vi "Calibration.vi"(8 "error in (no error)":errorcluster, 11 "Connection Data In":T1) -> (0 "error out":errorcluster={"status"=TRUE, "code"=1172, "source"="Constructor Node Error creating instance of Uri in assembly System.Uri, System, Version=4.0.0.0, Culture=neutral, PublicKeyToken=b77a5c561934e089, (System.UriFormatException: Invalid URI: The hostname could not be parsed.) <append><b>System.UriFormatException</b> in MSX-E3701_dll.lvlib:Connection Open.vi->MSX-E3701_dll.lvlib:Calibration.vi"}, 3 "Connection Data Out":T1)   [LabVIEW 2014, in "MSX-E3711_dll.lvlib"]
doc: "Paanel Frontal que permite la calibracion de transductores."
uses:
  MSX-E3711_dll.lvlib
  Typedef/Calibration Data.ctl
  Typedef/Connection Data.ctl
  E:/Repositorio Magnis/INF002/v0/Modules/HAL/Drivers/Sync/ADDI-DATA MSX-E3711/API/MSXE371x.dll
  MSXE371x.dll
  E:/Repositorio Magnis/INF002/v0/Modules/HAL/Drivers/Sync/ADDI-DATA MSX-E3711/API/MXCommon.dll
  MXCommon.dll
  Typedef/Calibration Enum.ctl
panel:
  out "ulChannel":u64
  in  "Transducer Selection":u64
  in  "Desired Position":dbl format="%#_g[mm]"
  in  "Stop":bool
  out "Progress Bar":u64(slide) scale=0.0..5.0
  out "Measured value":dbl format="%#_g[mm]"
  out "Indicator":string="Leyendo los transductores de la base de datos."
  in  "Next":bool
  in  "Start":bool
  out "Cluster Calibration":T2
  # "TRANSDUCER CALIBRATION"
  # "Progress Bar"
  # "Information"
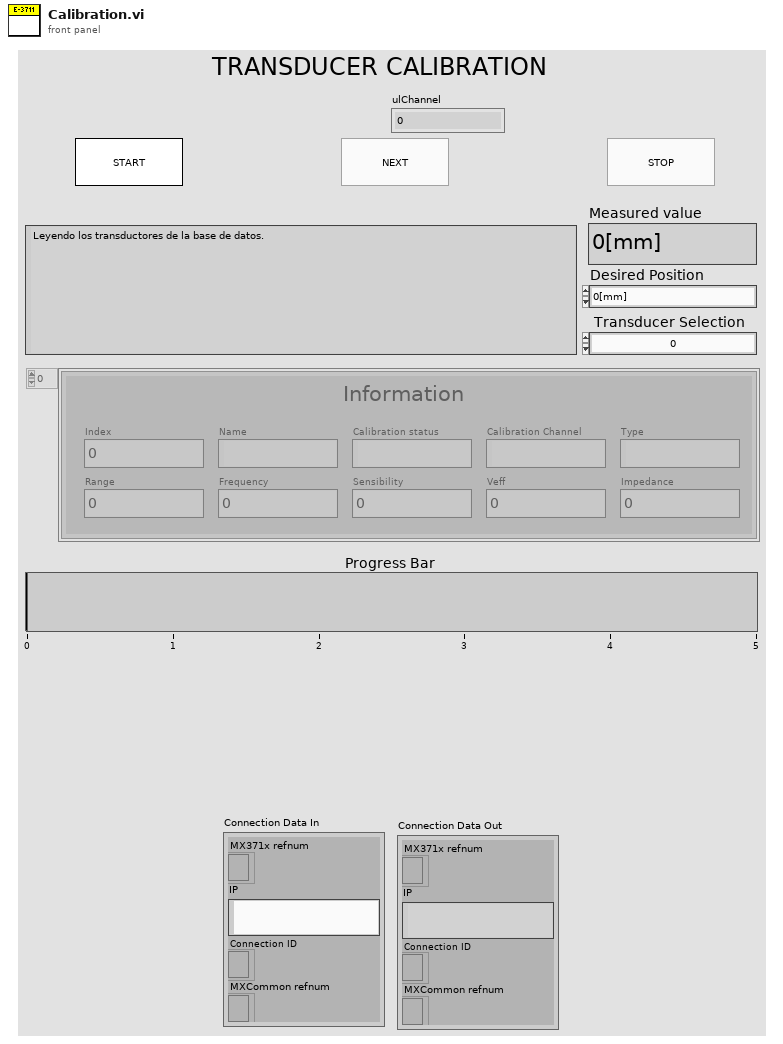
[diagram p1: front panel]
types:
  T1 = typedef "MSX-E3711_dll.lvlib/Connection Data.ctl" = cluster{"MX371x refnum":refnum<k24>, "IP":string, "Connection ID ":refnum<k5>, "MXCommon refnum":refnum<k24>}
  T2 = typedef "MSX-E3711_dll.lvlib/Calibration Data.ctl" = cluster{"Calibration status":string, "Name":string, "Index":u64, "Range":dbl, "Sensibility":dbl, "Veff":dbl, "Frequency":u64, "Impedance":u64, "Type":string, "Calibration Channel":string}[]
  T3 = typedef "MSX-E3711_dll.lvlib/Calibration Enum.ctl" = enum16{"Init", "Idle Start", "Idle Next", "Open Web Service", "Read Transducers", "StartCalibration", "CalibrationGetCurrentStatus", "Save or Omit", "Close Web Service", "Idle Final"}
  T4 = enum8{"Enabled", "Disabled", "Disabled and Grayed Out"}
  T5 = cluster{"Calibration status":string, "Name":string, "Index":u64, "Range":dbl, "Sensibility":dbl, "Veff":dbl, "Frequency":u64, "Impedance":u64, "Type":string, "Calibration Channel":string}
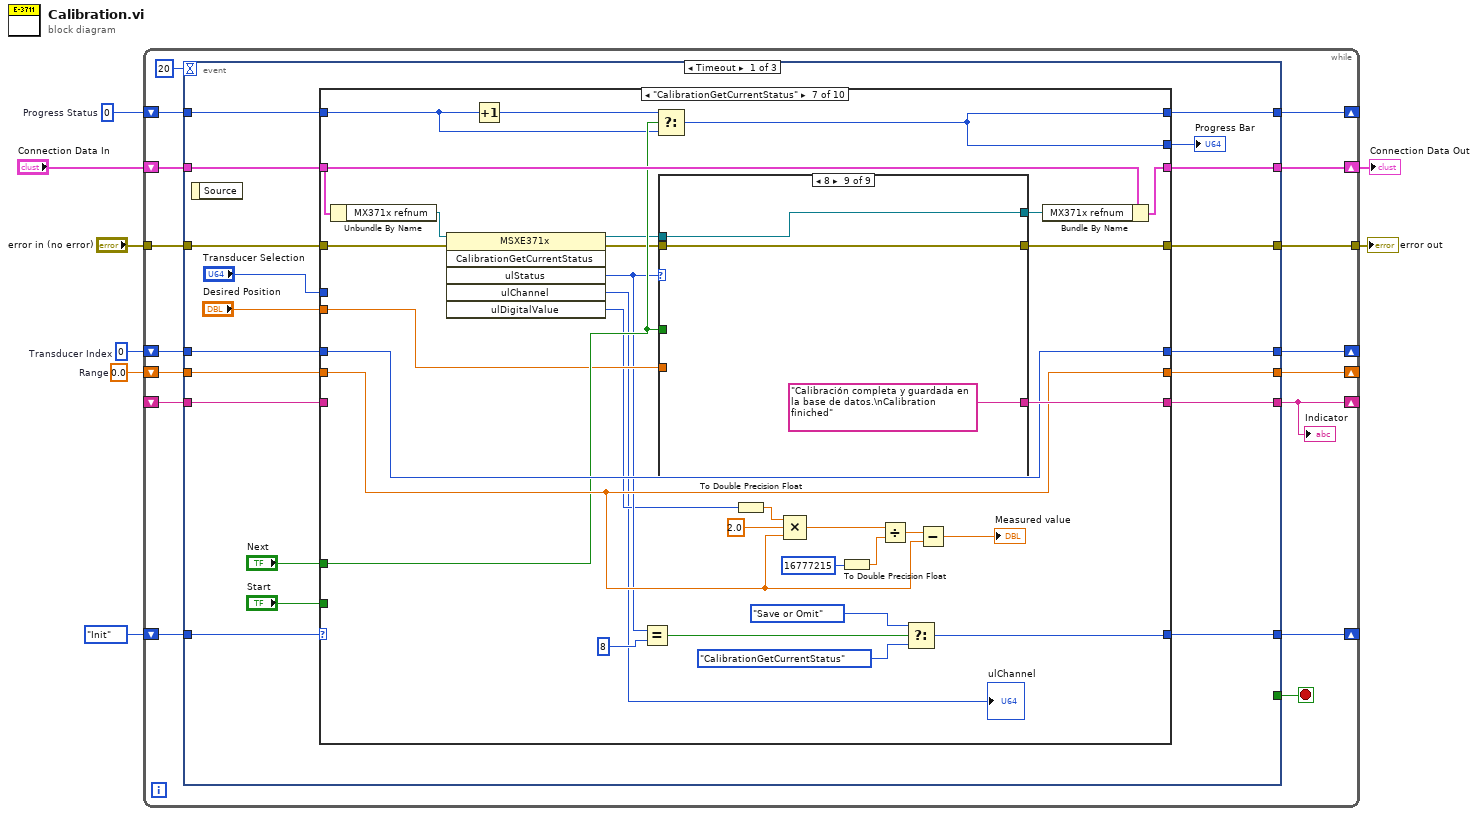
[diagram p0: block diagram]
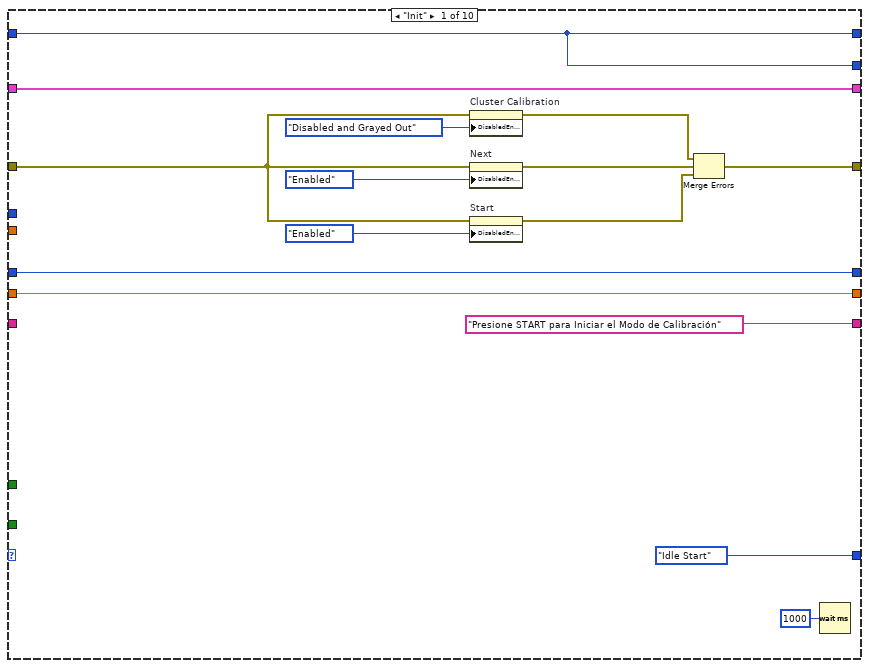
[diagram p2: hidden frame]
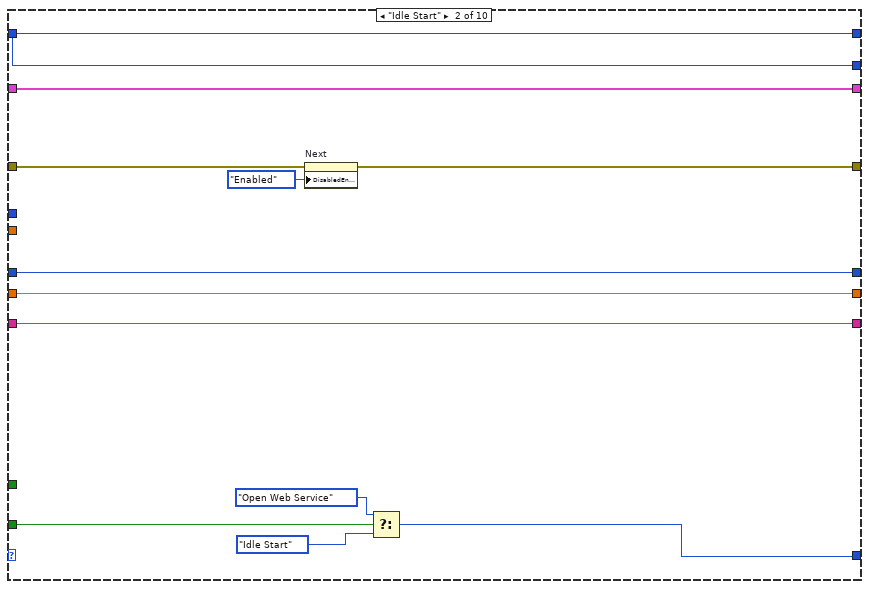
[diagram p3: hidden frame]
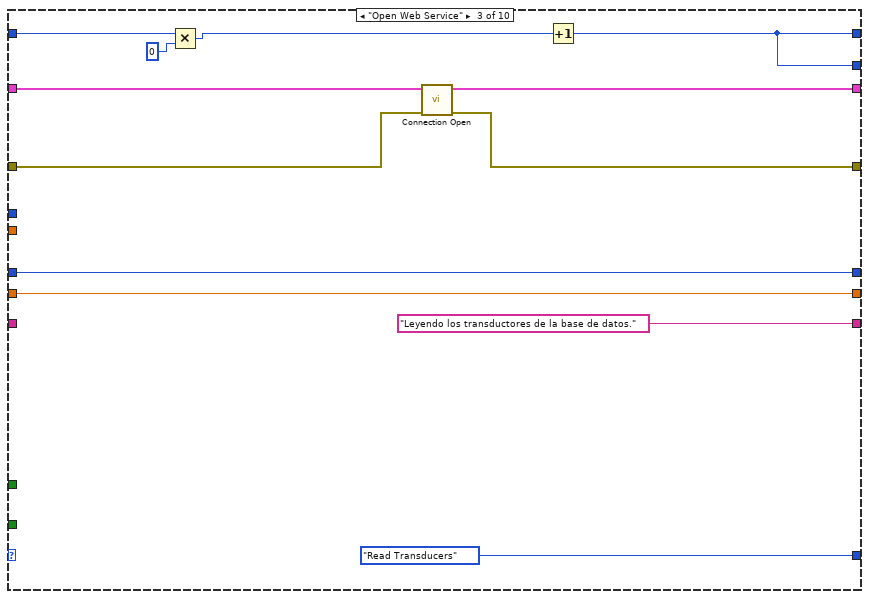
[diagram p4: hidden frame]
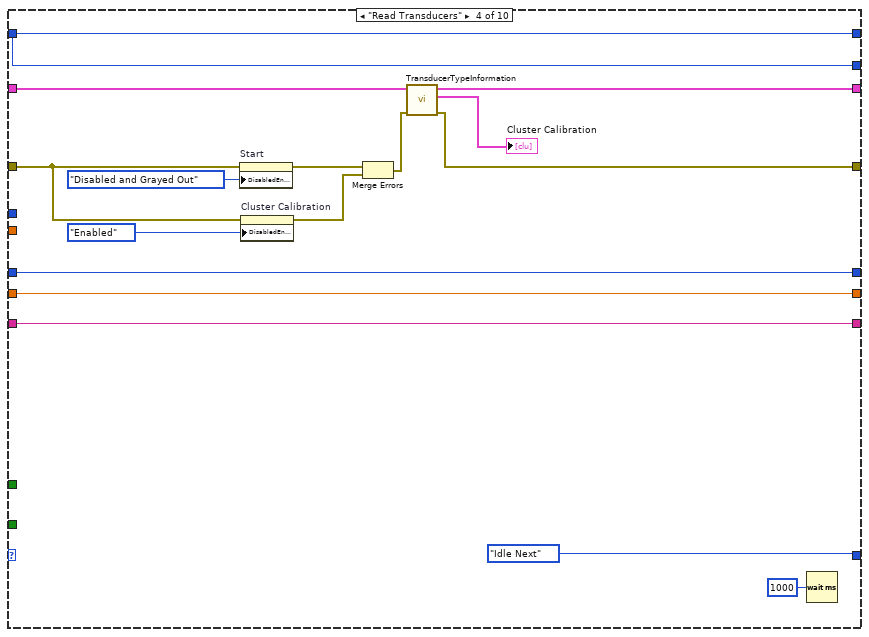
[diagram p5: hidden frame]
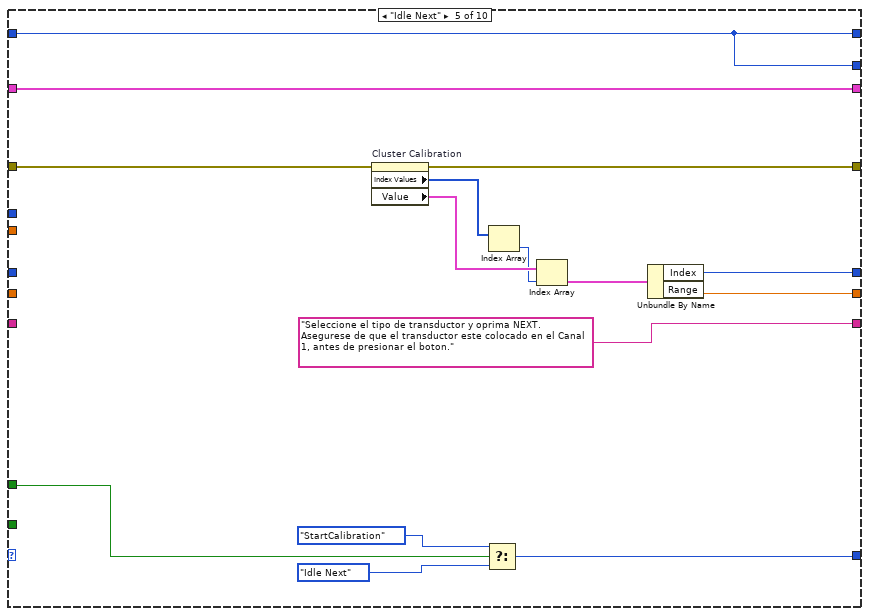
[diagram p6: hidden frame]
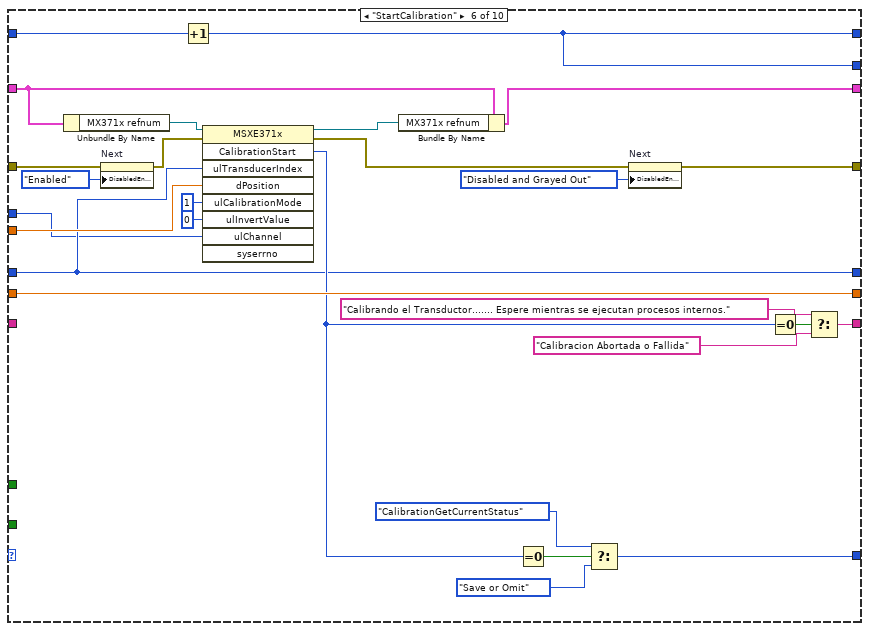
[diagram p7: hidden frame]
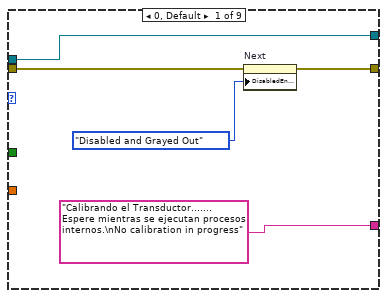
[diagram p8: hidden frame]
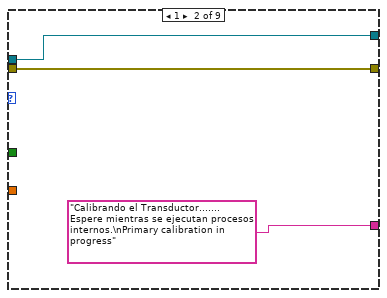
[diagram p9: hidden frame]
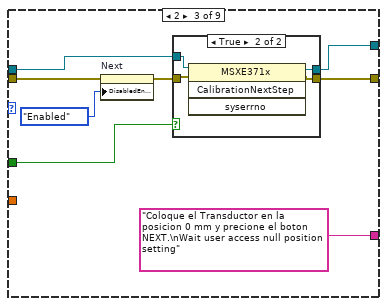
[diagram p10: hidden frame]
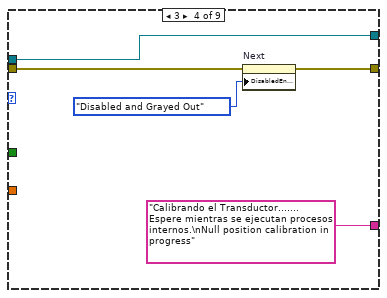
[diagram p12: hidden frame]
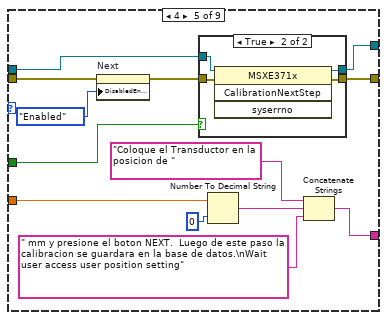
[diagram p13: hidden frame]
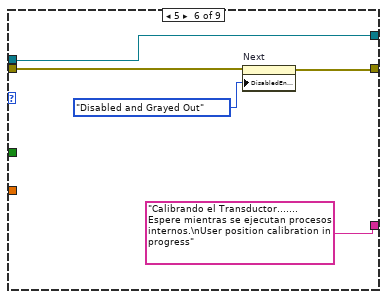
[diagram p15: hidden frame]
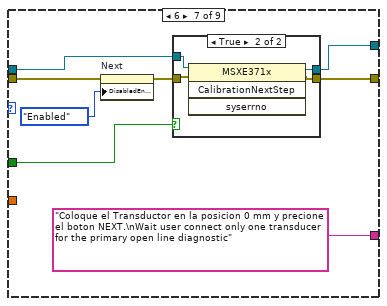
[diagram p16: hidden frame]
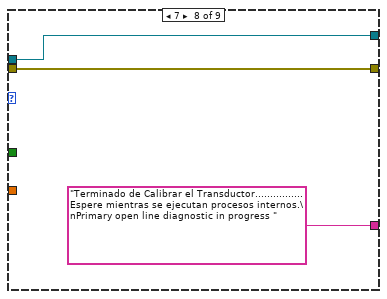
[diagram p18: hidden frame]
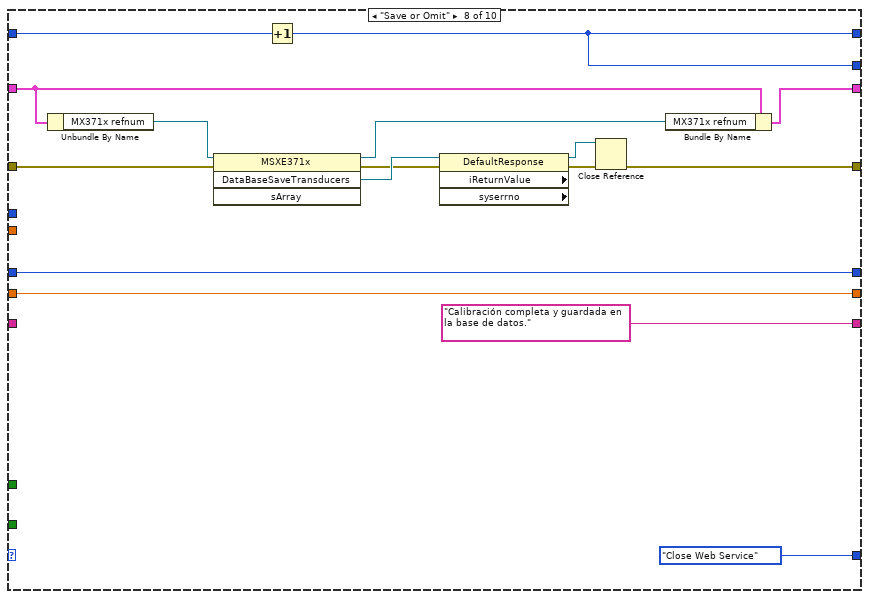
[diagram p19: hidden frame]
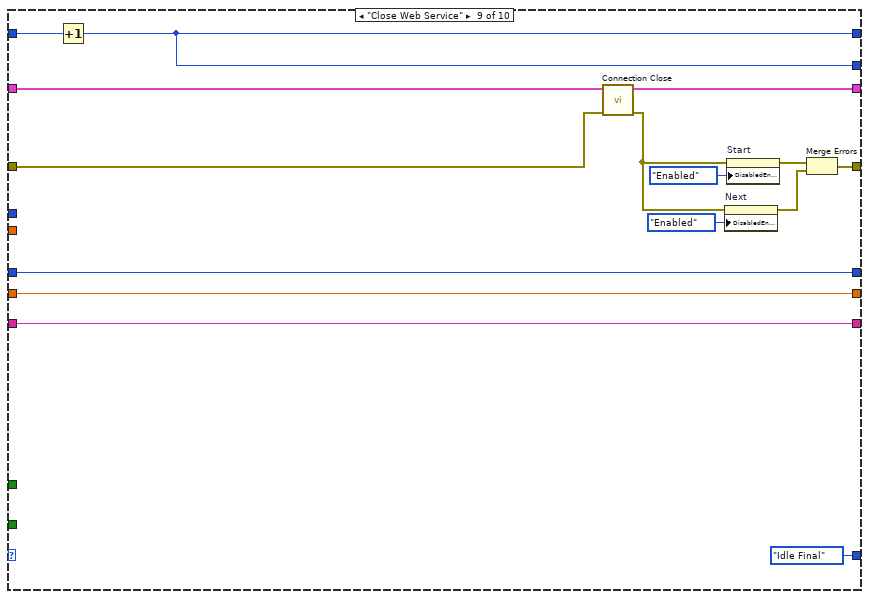
[diagram p20: hidden frame]
diagram:
  w3 = u64 0  # Progress Status
  w4 = 0.0  # Range
  w5 = u64 0  # Transducer Index
  n1 = while {
    tunnel: [w20] -> w8
    tunnel: "error in (no error)" -> [w22]
    shift-right: [w23] -> w1
    shift-left: "Connection Data In" -> [w24]
    shift-right: [w14] -> _
    shift-left: Calibration_Enum."Init" ("Enum") -> [w19]
    shift-right: [w18] -> _
    shift-left: w5 -> [w16]
    shift-right: [w17] -> _
    shift-left: w4 -> [w15]
    shift-right: [w12] -> _
    shift-left: w3 -> [w13]
    shift-right: [w10] -> _
    shift-left: _ -> [w9]
    stop <- w21 stop-if-true
    n2 = event shown="[0] Timeout" {
      selector: _ -> [_ _ _]
      dyn-events: _ -> [_ _ _]
      timeout: 20 -> [_ _ _]
      tunnel: w24 -> [w43 w293 w299]
      tunnel: [w42 w292 w298] -> w23
      tunnel: w22 -> [w41 w288 w297]
      tunnel: [_ _ w300] -> w21
      tunnel: [w40 w285 w296] -> w20
      tunnel: w19 -> [w38 _ _]
      tunnel: [w37 _ _] -> w18
      tunnel: [w36 _ _] -> w17
      tunnel: w16 -> [w35 _ _]
      tunnel: w15 -> [w34 _ _]
      tunnel: [w33 Calibration_Enum."Init" ("Enum") _] -> w14
      tunnel: w13 -> [w31 _ _]
      tunnel: [w30 u64 0 ("Progress Status") u64 0 ("Progress Status")] -> w12
      tunnel: [w28 "Calibracion Abortada o Fallida" ("Caption.Text") "ADIOS" ("Caption.Text")] -> w10
      tunnel: w9 -> [w27 _ _]
      event Timeout {
        n3 = event-data() -> ()  [unwired: 1 in, 1 out]
        n4 = case shown="\"CalibrationGetCurrentStatus\"" w38 {
          tunnel: w43 -> [w54 w70 w82 w98 w110 w140 w171 w258 w260 w284]
          tunnel: [w54 w70 w81 w97 w110 w139 w170 w257 w273 w284] -> w42
          tunnel: [w55 w61 w80 w96 w109 w125 w158 w256 w263 w283] -> w40
          tunnel: w41 -> [w50 w62 w79 w89 w100 w137 w147 w247 w259 w283]
          tunnel: [Calibration_Enum."Idle Start" ("Enum") w60 Calibration_Enum."Read Transducers" ("f") Calibration_Enum."Idle Next" ("Enum") w99 w124 w149 Calibration_Enum."Close Web Service" ("Enum") Calibration_Enum."Idle Final" ("Enum") w277] -> w33
          tunnel: "Start" -> [_ w68 _ _ _ _ _ _ _ w279]
          tunnel: [w48 w66 w78 w88 w102 w117 w154 w250 w271 w282] -> w37
          tunnel: [w47 w65 w77 w87 w107 w136 w155 w254 w270 w281] -> w36
          tunnel: w35 -> [w48 w66 w78 w88 _ w117 w154 w250 w271 w282]
          tunnel: w34 -> [w47 w65 w77 w87 _ w136 w155 w254 w270 w281]
          tunnel: ["Presione START para Iniciar el Modo de Calibración" ("Indicator") w59 "Leyendo los transductores de la base de datos." ("Indicator") w83 "Seleccione el tipo de transductor y oprima NEXT. Asegurese de que el transductor este colocado en el Canal 1, antes de presionar el boton." ("Caption.Text") w130 w156 "Calibración completa y guardada en la base de datos." ("Caption.Text") w261 w275] -> w28
          tunnel: "Next" -> [_ _ _ _ w103 _ w152 _ _ _]
          tunnel: [w46 w64 w75 w85 w101 w127 w153 w251 w262 w276] -> w30
          tunnel: w31 -> [w46 w64 w73 w85 w101 w128 w150 w252 w268 w276]
          tunnel: [w46 w64 w75 w85 w101 w127 w153 w251 w262 w276] -> w29
          tunnel: w27 -> [_ w59 _ w83 _ _ _ _ w261 w275]
          tunnel: "Desired Position" -> [_ _ _ _ _ w118 w148 _ _ _]
          tunnel: "Transducer Selection" -> [_ _ _ _ _ w116 _ _ _ _]
          frame "Init" {
            n5 = property on="Cluster Calibration" class="Arr (strict)"(error in=w50, "DisabledEnum"=T4."Disabled and Grayed Out" ("Disabled")) -> (error out=w56:errorcluster)  [unwired: 1 in, 1 out]
            n6 = property on="Next" class="Bool"(error in=w50, "DisabledEnum"=T4."Enabled" ("Disabled")) -> (error out=w52:errorcluster)  [unwired: 1 in, 1 out]
            n7 = property on="Start" class="Bool"(error in=w50, "DisabledEnum"=T4."Enabled" ("Disabled")) -> (error out=w51:errorcluster)  [unwired: 1 in, 1 out]
            n8 = Merge Errors(w56, w52, w51) -> (w55:errorcluster)
            n9 = Wait (ms)(milliseconds to wait=u32 1000) -> ()  [unwired: 1 out]
          }
          frame "Idle Start" {
            n10 = property on="Next" class="Bool"(error in=w62, "DisabledEnum"=T4."Enabled" ("Disabled")) -> (error out=w61:errorcluster)  [unwired: 1 in, 1 out]
            n11 = Select(t=Calibration_Enum."Open Web Service" ("Enum"), s=w68, f=Calibration_Enum."Idle Start") -> (s? t:f=w60:T3)
          }
          frame "Open Web Service" {
            n12 = Multiply(x=w73, y=u64 0) -> (x*y=w74:u64)
            n13 = call "Connection Open.vi"("error in (no error)"=w79, "Connection Data In"=w82) -> ("error out"=w80:errorcluster, "Connection Data Out"=w81:T1)  [unwired: 8 in]
            n14 = Increment(x=w74) -> (x+1=w75:u64)
          }
          frame "Read Transducers" {
            n15 = property on="Start" class="Bool"(error in=w89, "DisabledEnum"=T4."Disabled and Grayed Out" ("Disabled")) -> (error out=w92:errorcluster)  [unwired: 1 in, 1 out]
            n16 = property on="Cluster Calibration" class="Arr (strict)"(error in=w89, "DisabledEnum"=T4."Enabled" ("Disabled")) -> (error out=w91:errorcluster)  [unwired: 1 in, 1 out]
            n17 = Merge Errors(w92, w91) -> (w90:errorcluster)
            n18 = call "TransducerTypeInformation.vi"("error in (no error)"=w90, "Connection Data In"=w98) -> ("error out"=w96:errorcluster, "Cluster Calibration"=→"Cluster Calibration":T2, "Connection Data Out"=w97:T1)  [unwired: 7 in]
            n19 = Wait (ms)(milliseconds to wait=u32 1000) -> ()  [unwired: 1 out]
          }
          frame "Idle Next" {
            n20 = property on="Cluster Calibration" class="Arr (strict)"(error in=w100) -> (error out=w109:errorcluster, "Index Values"=w113:u32[], "Value"=w112:T2)  [unwired: 1 in, 1 out]
            n21 = Select(t=Calibration_Enum."StartCalibration" ("Enum"), s=w103, f=Calibration_Enum."Idle Next") -> (s? t:f=w99:T3)
            n22 = Index Array(array=w113) -> (element=w108:u32)  [unwired: 1 in]
            n23 = Index Array(array=w112, index=w108) -> (element=w111:T5)
            n24 = Unbundle By Name(w111) -> ("Index"=w102:u64, "Range"=w107:dbl)
          }
          frame "StartCalibration" {
            n25 = Unbundle By Name(w140) -> ("MX371x refnum"=w123:refnum<k24>)
            n26 = property on="Next" class="Bool"(error in=w137, "DisabledEnum"=T4."Enabled" ("Disabled")) -> (error out=w122:errorcluster)  [unwired: 1 in, 1 out]
            n27 = Increment(x=w128) -> (x+1=w127:u64)
            n28 = invoke class="MSXE371x" method="CalibrationStart"(reference=w123, error in=w122, "ulTransducerIndex"=w117, "dPosition"=w118, "ulCalibrationMode"=u64 1, "ulInvertValue"=u64 0, "ulChannel"=w116) -> (reference out=w120:refnum<k24>, error out=w121:errorcluster, "CalibrationStart"=w119:i32)  [unwired: 2 in, 6 out]
            n29 = Bundle By Name(cluster=w140, "MX371x refnum"=w120) -> (w139:T1)
            n30 = Equal To 0?(x=w119) -> (x = 0?=w135:bool)
            n31 = Select(t=Calibration_Enum."CalibrationGetCurrentStatus" ("Enum"), s=w135, f=Calibration_Enum."Save or Omit" ("Enum")) -> (s? t:f=w124:T3)
            n32 = property on="Next" class="Bool"(error in=w121, "DisabledEnum"=T4."Disabled and Grayed Out" ("Disabled")) -> (error out=w125:errorcluster)  [unwired: 1 in, 1 out]
            n33 = Equal To 0?(x=w119) -> (x = 0?=w132:bool)
            n34 = Select(t="Calibrando el Transductor....... Espere mientras se ejecutan procesos internos." ("Caption.Text"), s=w132, f="Calibracion Abortada o Fallida") -> (s? t:f=w130:string)
          }
          frame "CalibrationGetCurrentStatus" {
            n35 = Unbundle By Name(w171) -> ("MX371x refnum"=w146:refnum<k24>)
            n36 = invoke class="MSXE371x" method="CalibrationGetCurrentStatus"(reference=w146, error in=w147) -> (reference out=w145:refnum<k24>, error out=w144:errorcluster, "ulStatus"=w143:u64, "ulChannel"=→"ulChannel":u64, "ulDigitalValue"=w142:u64)  [unwired: 4 in, 1 out]
            n37 = Increment(x=w150) -> (x+1=w151:u64)
            n38 = Equal?(x=w143, y=u64 8) -> (x = y?=w161:bool)
            n39 = Select(t=w151, s=w152, f=w150) -> (s? t:f=w153:u64)
            n40 = case shown="8" w143 {
              tunnel: w144 -> [w175 w179 w182 w197 w207 w221 w227 w239 w240]
              tunnel: w145 -> [w173 w178 w183 w194 w208 w219 w228 w238 w242]
              tunnel: [w174 w179 w187 w196 w206 w220 w223 w239 w240] -> w158
              tunnel: [w173 w178 w186 w194 w200 w219 w225 w238 w242] -> w157
              tunnel: ["Calibrando el Transductor....... Espere mientras se ejecutan procesos internos.\nNo calibration in progress" ("Caption.Text") "Calibrando el Transductor....... Espere mientras se ejecutan procesos internos.\nPrimary calibration in progress" ("Caption.Text") "Coloque el Transductor en la posicion 0 mm y precione el boton NEXT.\nWait user access null position setting" ("Caption.Text") "Calibrando el Transductor....... Espere mientras se ejecutan procesos internos.\nNull position calibration in progress" ("Caption.Text") w201 "Calibrando el Transductor....... Espere mientras se ejecutan procesos internos.\nUser position calibration in progress" ("Caption.Text") "Coloque el Transductor en la posicion 0 mm y precione el boton NEXT.\nWait user connect only one transducer for the primary open line diagnostic" ("Caption.Text") "Terminado de Calibrar el Transductor................ Espere mientras se ejecutan procesos internos.\nPrimary open line diagnostic in progress " ("Caption.Text") "Calibración completa y guardada en la base de datos.\nCalibration finiched" ("Caption.Text")] -> w156
              tunnel: w152 -> [_ _ w180 _ w209 _ w226 _ _]
              tunnel: w148 -> [_ _ _ _ w199 _ _ _ _]
              frame 0, Default {
                n41 = property on="Next" class="Bool"(error in=w175, "DisabledEnum"=T4."Disabled and Grayed Out" ("Disabled")) -> (error out=w174:errorcluster)  [unwired: 1 in, 1 out]
              }
              frame 1 {
              }
              frame 2 {
                n42 = property on="Next" class="Bool"(error in=w182, "DisabledEnum"=T4."Enabled" ("Disabled")) -> (error out=w184:errorcluster)  [unwired: 1 in, 1 out]
                n43 = case shown="True" w180 {
                  tunnel: [w188 w192] -> w187
                  tunnel: [w189 w193] -> w186
                  tunnel: w184 -> [w188 w191]
                  tunnel: w183 -> [w189 w190]
                  frame False {
                  }
                  frame True {
                    n44 = invoke class="MSXE371x" method="CalibrationNextStep"(reference=w190, error in=w191) -> (reference out=w193:refnum<k24>, error out=w192:errorcluster)  [unwired: 2 in, 2 out]
                  }
                }
              }
              frame 3 {
                n45 = property on="Next" class="Bool"(error in=w197, "DisabledEnum"=T4."Disabled and Grayed Out" ("Disabled")) -> (error out=w196:errorcluster)  [unwired: 1 in, 1 out]
              }
              frame 4 {
                n46 = property on="Next" class="Bool"(error in=w207, "DisabledEnum"=T4."Enabled" ("Disabled")) -> (error out=w211:errorcluster)  [unwired: 1 in, 1 out]
                n47 = case shown="True" w209 {
                  tunnel: [w212 w214] -> w206
                  tunnel: [w213 w215] -> w200
                  tunnel: w211 -> [w212 w216]
                  tunnel: w208 -> [w213 w217]
                  frame False {
                  }
                  frame True {
                    n48 = invoke class="MSXE371x" method="CalibrationNextStep"(reference=w217, error in=w216) -> (reference out=w215:refnum<k24>, error out=w214:errorcluster)  [unwired: 2 in, 2 out]
                  }
                }
                n49 = Number To Decimal String(number=w199, width (-)=i16 0) -> (decimal integer string=w204:string)
                n50 = Concatenate Strings("Coloque el Transductor en la posicion de " ("Caption.Text"), w204, " mm y presione el boton NEXT.  Luego de este paso la calibracion se guardara en la base de datos.\nWait user access user position setting") -> (w201:string)
              }
              frame 5 {
                n51 = property on="Next" class="Bool"(error in=w221, "DisabledEnum"=T4."Disabled and Grayed Out" ("Disabled")) -> (error out=w220:errorcluster)  [unwired: 1 in, 1 out]
              }
              frame 6 {
                n52 = property on="Next" class="Bool"(error in=w227, "DisabledEnum"=T4."Enabled" ("Disabled")) -> (error out=w230:errorcluster)  [unwired: 1 in, 1 out]
                n53 = case shown="True" w226 {
                  tunnel: [w231 w235] -> w223
                  tunnel: [w232 w236] -> w225
                  tunnel: w230 -> [w231 w234]
                  tunnel: w228 -> [w232 w233]
                  frame False {
                  }
                  frame True {
                    n54 = invoke class="MSXE371x" method="CalibrationNextStep"(reference=w233, error in=w234) -> (reference out=w236:refnum<k24>, error out=w235:errorcluster)  [unwired: 2 in, 2 out]
                  }
                }
              }
              frame 7 {
              }
              frame 8 {
              }
            }
            n55 = To Double Precision Float(number=w142) -> (double precision float=w165:dbl)
            n56 = Compound Arithmetic op=MULTIPLY(w165, 2.0 ("x"), w155) -> (w166:dbl)
            n57 = To Double Precision Float(number=u64 16777215 ("x")) -> (double precision float=w163:dbl)
            n58 = Divide(x=w166, y=w163) -> (x/y=w167:dbl)
            n59 = Select(t=Calibration_Enum."Save or Omit" ("Enum"), s=w161, f=Calibration_Enum."CalibrationGetCurrentStatus" ("Enum")) -> (s? t:f=w149:T3)
            n60 = Subtract(x=w167, y=w155) -> (x-y=→"Measured value":dbl)
            n61 = Bundle By Name(cluster=w171, "MX371x refnum"=w157) -> (w170:T1)
          }
          frame "Save or Omit" {
            n62 = Unbundle By Name(w258) -> ("MX371x refnum"=w249:refnum<k24>)
            n63 = invoke class="MSXE371x" method="DataBaseSaveTransducers"(reference=w249, error in=w247) -> (reference out=w248:refnum<k24>, error out=w245:errorcluster, "DataBaseSaveTransducers"=w246:refnum<k24>)  [unwired: 2 in, 1 out]
            n64 = Increment(x=w252) -> (x+1=w251:u64)
            n65 = property class="DefaultResponse" props=["iReturnValue", "syserrno"](reference=w246, error in=w245) -> (reference out=w244:refnum<k24>, error out=w243:errorcluster)  [unwired: 2 out]
            n66 = Close Reference(reference=w244, error in (no error)=w243) -> (error out=w256:errorcluster)
            n67 = Bundle By Name(cluster=w258, "MX371x refnum"=w248) -> (w257:T1)
          }
          frame "Close Web Service" {
            n68 = Increment(x=w268) -> (x+1=w262:u64)
            n69 = call "Connection Close.vi"("error in (no error)"=w259, "Connection Data In"=w260) -> ("error out"=w266:errorcluster, "Connection Data Out"=w273:T1)  [unwired: 8 in]
            n70 = property on="Next" class="Bool"(error in=w266, "DisabledEnum"=T4."Enabled" ("Disabled")) -> (error out=w265:errorcluster)  [unwired: 1 in, 1 out]
            n71 = property on="Start" class="Bool"(error in=w266, "DisabledEnum"=T4."Enabled" ("Disabled")) -> (error out=w264:errorcluster)  [unwired: 1 in, 1 out]
            n72 = Merge Errors(w264, w265) -> (w263:errorcluster)
          }
          frame "Idle Final" {
            n73 = Select(t=Calibration_Enum."Open Web Service", s=w279, f=Calibration_Enum."Idle Final" ("Enum")) -> (s? t:f=w277:T3)
            n74 = Wait (ms)(milliseconds to wait=u32 1000) -> ()  [unwired: 1 out]
          }
        }
        "Progress Bar" <- w29
      }
      event "Stop": Value Change {
        n75 = event-data() -> ()  [unwired: 1 in, 1 out]
        n76 = Unbundle By Name(w293) -> ("MX371x refnum"=w287:refnum<k24>)
        n77 = invoke class="MSXE371x" method="CalibrationBreak"(reference=w287, error in=w288) -> (reference out=w286:refnum<k24>, error out=w285:errorcluster)  [unwired: 2 in, 2 out]
        n78 = Bundle By Name(cluster=w293, "MX371x refnum"=w286) -> (w292:T1)
      }
      event Panel Close? {
        n79 = event-data() -> ()  [unwired: 1 in, 4 out]
        n80 = call "Connection Close.vi"("error in (no error)"=w297, "Connection Data In"=w299) -> ("error out"=w296:errorcluster, "Connection Data Out"=w298:T1)  [unwired: 8 in]
        n81 = Or(x=w296, y=TRUE) -> (x .or. y?=w300:bool)
        n82 = event-data("Discard?"=FALSE) -> ()  [unwired: 1 in, 1 out]
      }
    }
    "Indicator" <- w10
  }
  "error out" <- w8
  "Connection Data Out" <- w1
